vi "_PC_Pub pingRT.vi"(0 "IPV4":string="100.100.0.123", 1 "items":i32=5) -> (2 "valid":bool)   [LabVIEW 2018]
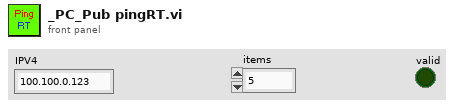
[diagram p1: front panel]
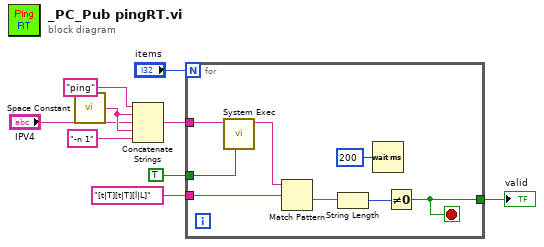
[diagram p0: block diagram]
diagram:
  n1 = call <vilib>:"Space Constant.vi"() -> ("String"=w8:string)
  n2 = Concatenate Strings("ping", w8, "IPV4", w8, "-n 1" ("string")) -> (w9:string)
  n3 = for {
    N: "items" -> [_]
    tunnel: w9 -> [w17]
    tunnel: TRUE ("run minimized? (F)") -> [w16]
    tunnel: "[t|T][t|T][l|L]" ("regular expression") -> [w15]
    tunnel: [w11] -> w1
    stop <- w11 stop-if-true
    n4 = call <vilib>:"System Exec.vi"("run minimized? (F)"=w16, "command line"=w17) -> ("standard output"=w14:string)  [unwired: 6 in, 3 out]
    n5 = Match Pattern(string=w14, regular expression=w15) -> (after substring=w12:string)  [unwired: 1 in, 3 out]
    n6 = String Length(string=w12) -> (length=w13:i32)
    n7 = Wait (ms)(milliseconds to wait=u32 200) -> ()  [unwired: 1 out]
    n8 = Not Equal To 0?(x=w13) -> (x != 0?=w11:bool)
  }
  "valid" <- w1
